vi "SDSU_DacParseHWRequest.vi"(10 "requested value":string) -> (0 "regs request":string, 1 "last reg":i32, 2 "first reg":i32, 3 "name out":string, 5 "partial?":bool)   [LabVIEW 2016]
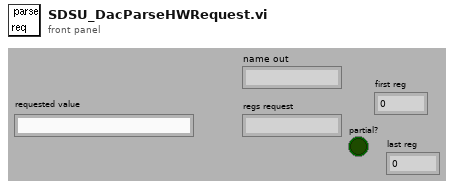
[diagram p1: front panel]
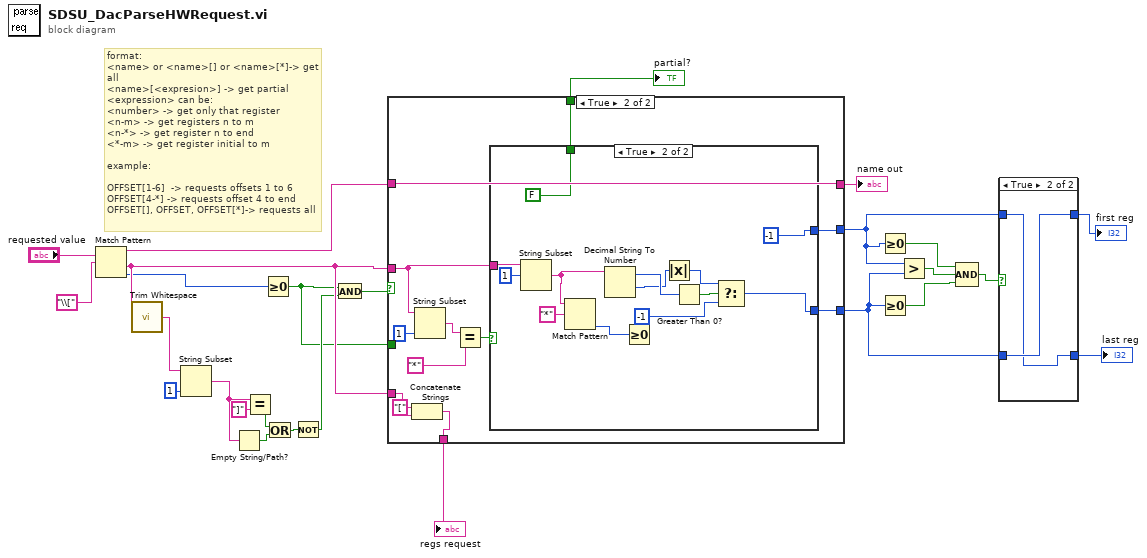
[diagram p0: block diagram]
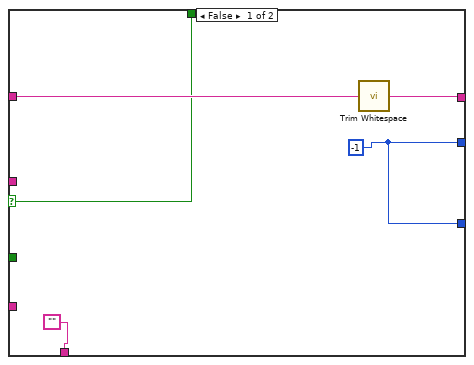
[diagram p3: hidden frame]
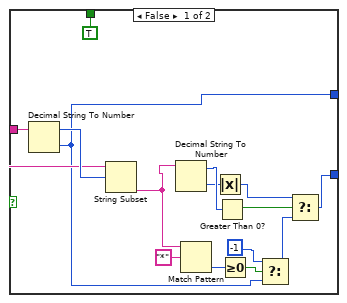
[diagram p4: hidden frame]
diagram:
  # "format:\n<name> or <name>[] or <name>[*]-> get all\n<name>[<expresion>] -> get partial\n<expression> can be:\n<number> -> get only that register\n<n-m> -> get registers n to m\n<n-*> -> get register n to end\n<*-m> -> get register initial to m\n\nexample:\n\nOFFSET[1-6]  -> requests offsets 1 to 6\nOFFSET[4-*] -> requests offset 4 to end\nOFFSET[], OFFSET, OFFSET[*]-> requests all"
  n1 = Match Pattern(string="requested value", regular expression="\\[") -> (before substring=w24:string, after substring=w13:string, offset past match=w3:i32)  [unwired: 2 out]
  n2 = call <vilib>:"Trim Whitespace.vi"("string"=w13) -> ("trimmed string"=w12:string)  [unwired: 1 in]
  n3 = String Subset(string=w12, length (rest)=1 ("length (rest)")) -> (substring=w9:string)  [unwired: 1 out]
  n4 = Empty String/Path?(string/path=w9) -> (empty?=w8:bool)
  n5 = Equal?(x=w9, y="]") -> (x = y?=w7:bool)
  n6 = Greater Or Equal To 0?(x=w3) -> (x >= 0?=w2:bool)
  n7 = Or(x=w7, y=w8) -> (x .or. y?=w4:bool)
  n8 = Not(x=w4) -> (.not. x?=w5:bool)
  n9 = And(x=w2, y=w5) -> (x .and. y?=w6:bool)
  n10 = case shown="True" w6 {
    selector: w6 -> [w27 _]
    tunnel: [w31 w37] -> w16
    tunnel: [w31 w42] -> w18
    tunnel: w13 -> [_ w38]
    tunnel: w24 -> [w29 w43]
    tunnel: [w30 w43] -> w23
    tunnel: w13 -> [_ w35]
    tunnel: ["" w34] -> w14
    tunnel: w2 -> [_ _]
    tunnel: [w27 w32] -> w1
    frame False {
      w31 = -1
      n11 = call <vilib>:"Trim Whitespace.vi"("string"=w29) -> ("trimmed string"=w30:string)  [unwired: 1 in]
    }
    frame True {
      n12 = Concatenate Strings("[" ("string"), w35) -> (w34:string)
      n13 = String Subset(string=w38, length (rest)=1 ("length (rest)")) -> (substring=w40:string)  [unwired: 1 out]
      n14 = Equal?(x=w40, y="*") -> (x = y?=w36:bool)
      n15 = case shown="True" w36 {
        tunnel: [w54 w64] -> w42
        tunnel: w38 -> [w47 w70]
        tunnel: [w45 -1 ("t")] -> w37
        tunnel: [TRUE ("partial?") FALSE ("partial?")] -> w32
        frame False {
          n16 = Decimal String To Number(string=w47) -> (offset past number=w58:i32, number=w45:i32)  [unwired: 2 out]
          n17 = String Subset(string=w47, offset (0)=w58) -> (substring=w46:string)  [unwired: 1 out]
          n18 = Decimal String To Number(string=w46) -> (offset past number=w56:i32, number=w55:i32)  [unwired: 2 out]
          n19 = Match Pattern(string=w46, regular expression="*") -> (offset past match=w51:i32)  [unwired: 4 out]
          n20 = Absolute Value(x=w55) -> (abs(x)=w52:i32)
          n21 = Greater Than 0?(x=w56) -> (x > 0?=w57:bool)
          n22 = Greater Or Equal To 0?(x=w51) -> (x >= 0?=w50:bool)
          n23 = Select(t=-1 ("f"), s=w50, f=w45) -> (s? t:f=w48:i32)
          n24 = Select(t=w52, s=w57, f=w48) -> (s? t:f=w54:i32)
        }
        frame True {
          n25 = String Subset(string=w70, offset (0)=1) -> (substring=w67:string)  [unwired: 1 out]
          n26 = Match Pattern(string=w67, regular expression="*") -> (offset past match=w63:i32)  [unwired: 4 out]
          n27 = Decimal String To Number(string=w67) -> (offset past number=w61:i32, number=w60:i32)  [unwired: 2 out]
          n28 = Greater Or Equal To 0?(x=w63) -> ()  [unwired: 1 out]
          n29 = Absolute Value(x=w60) -> (abs(x)=w65:i32)
          n30 = Greater Than 0?(x=w61) -> (x > 0?=w66:bool)
          n31 = Select(t=w65, s=w66, f=-1 ("t")) -> (s? t:f=w64:i32)
        }
      }
    }
  }
  "name out" <- w23
  "regs request" <- w14
  "partial?" <- w1
  n32 = Greater Or Equal To 0?(x=w16) -> (x >= 0?=w22:bool)
  n33 = Greater Or Equal To 0?(x=w18) -> (x >= 0?=w20:bool)
  n34 = Greater?(x=w16, y=w18) -> (0:w21:bool)
  n35 = Compound Arithmetic op=AND(w22, w21, w20) -> (w19:bool)
  n36 = case shown="True" w19 {
    tunnel: w18 -> [w73 w75]
    tunnel: [w73 w74] -> w17
    tunnel: w16 -> [w72 w74]
    tunnel: [w72 w75] -> w15
    frame False {
    }
    frame True {
    }
  }
  "first reg" <- w15
  "last reg" <- w17
